vi "New Text Log File.vi"(4 "Header Text (\"\")":string, 6 "Decimal Places (3)":u32=3, 7 "Delimiter (Tab)":T1, 8 "error in (no error)":errorcluster, 9 "Channel Paths":T2[](array[typedef]), 10 "File Conflict Operation":T4, 11 "Log File Path":path) -> (0 "error out":errorcluster, 3 "TextLogFile Ref":T3)   [LabVIEW 2020, in "NI_VS Data Logging API.lvlib"]
uses:
  <vilib>/NI VeriStand/Execution/DataLogging/NI_VS Data Logging API.lvlib
  <vilib>/NI VeriStand/Execution/DataLogging/File Conflict Operation.ctl
  <vilib>/NI VeriStand/Execution/DataLogging/TextLogFile Ref.ctl
  NationalInstruments.VeriStand.ClientAPI
  <vilib>/NI VeriStand/Execution/DataLogging/Text Channel.ctl
  <vilib>/NI VeriStand/Execution/DataLogging/Delimiter.ctl
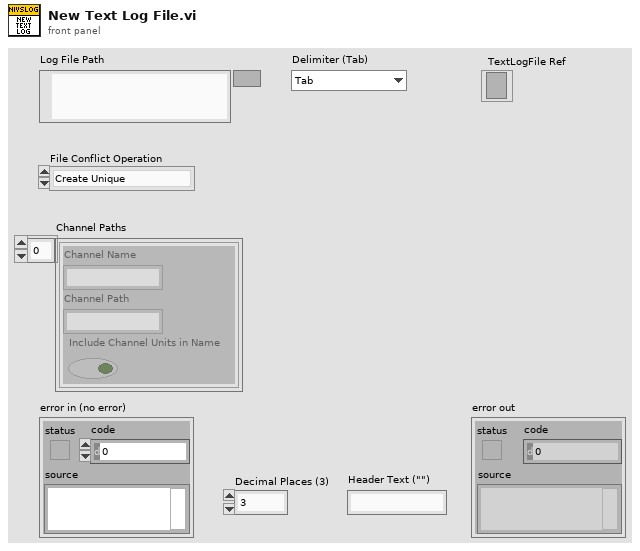
[diagram p1: front panel]
types:
  T1 = typedef "NI_VS Data Logging API.lvlib/Delimiter.ctl" = enum16{"Tab", "Comma"}
  T2 = typedef "NI_VS Data Logging API.lvlib/Text Channel.ctl" = cluster{"Channel Name":string, "Channel Path":string, "Include Channel Units in Name":bool}
  T3 = typedef "NI_VS Data Logging API.lvlib/TextLogFile Ref.ctl" = refnum<k24>
  T4 = typedef "NI_VS Data Logging API.lvlib/File Conflict Operation.ctl" = enum16{"Create Unique", "Append to Existing", "Overwrite"}
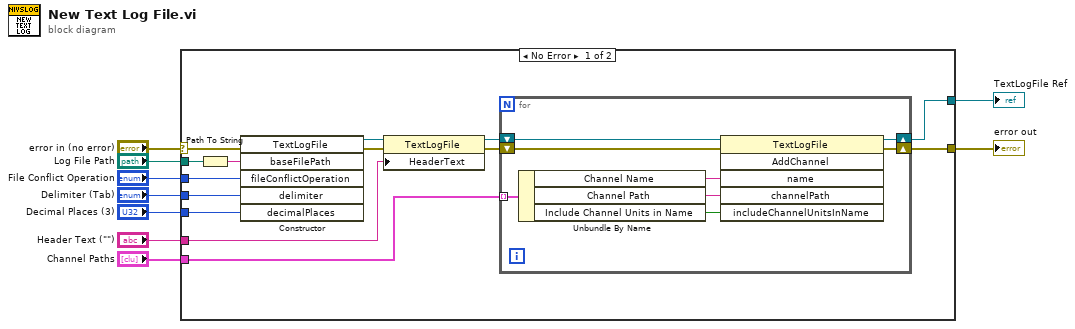
[diagram p0: block diagram]
diagram:
  n1 = case shown="No Error" "error in (no error)" {
    selector: "error in (no error)" -> [w18 w32]
    tunnel: "Decimal Places (3)" -> [w23 _]
    tunnel: "File Conflict Operation" -> [w22 _]
    tunnel: "Log File Path" -> [w21 _]
    tunnel: "Delimiter (Tab)" -> [w19 _]
    tunnel: [w16 w32] -> w5
    tunnel: "Channel Paths" -> [w17 _]
    tunnel: [w15 _] -> w2
    tunnel: "Header Text (\"\")" -> [w10 _]
    frame No Error {
      n2 = Path To String(path=w21) -> (string=w20:string)
      n3 = constructor class="TextLogFile"(error in=w18, "baseFilePath"=w20, "fileConflictOperation"=w22, "delimiter"=w19, "decimalPlaces"=w23) -> (reference out=w13:refnum<k24>, error out=w14:errorcluster)  [unwired: 2 in, 5 out]
      n4 = property class="TextLogFile"(reference=w13, error in=w14, "HeaderText"=w10) -> (reference out=w12:refnum<k24>, error out=w11:errorcluster)
      n5 = for {
        tunnel: w17 -> [w27] mode=indexing
        shift-right: [w29] -> w15
        shift-left: w12 -> [w31]
        shift-right: [w28] -> w16
        shift-left: w11 -> [w30]
        n6 = Unbundle By Name(w27) -> ("Channel Name"=w26:string, "Channel Path"=w25:string, "Include Channel Units in Name"=w24:bool)
        n7 = invoke class="TextLogFile" method="AddChannel"(reference=w31, error in=w30, "name"=w26, "channelPath"=w25, "includeChannelUnitsInName"=w24) -> (reference out=w29:refnum<k24>, error out=w28:errorcluster)  [unwired: 1 in, 4 out]
      }
    }
    frame Error {
    }
  }
  "TextLogFile Ref" <- w2
  "error out" <- w5
